vi "DynamixelUnitsToTorque.vi"(11 "Dynamixel Value":dbl) -> (3 "Torque on Dynamixel (N*m)":dbl)   [LabVIEW 2013]
doc: "This VI should take the output of the Dynamixel torque read (in some form of %, I believe) and turn it into torque ith actual units (N*m). The transfer will have to be determined experimentally.\n\nEric Schneider, March 2014"
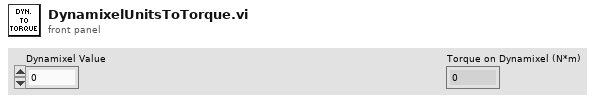
[diagram p1: front panel]
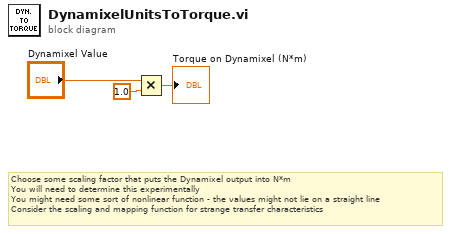
[diagram p0: block diagram]
diagram:
  # "Choose some scaling factor that puts the Dynamixel output into N*m\nYou will need to determine this experimentally\nYou might need some sort of nonlinear function - the values might not lie on a straight line\nConsider the scaling and mapping function for strange transfer characteristics"
  n1 = Multiply(x="Dynamixel Value", y=1.0) -> (x*y=→"Torque on Dynamixel (N*m)":dbl)
